vi "pump_test_backup.vi"() -> ()   [LabVIEW 2019]
uses:
  <vilib>/Instr/_visa.llb/VISA Configure Serial Port (Instr).vi
panel:
  in  "Frequency (%)":u16
  out "Error Out":errorcluster={"status"=FALSE, "code"=1073676294, "source"="VISA Read in pump_test.vi"}
  out "Time and torque":string="15.07.22\t0\r"
  in  "stop":bool
  out "Current readind (A)":dbl format="%.2g"
  out "Frequency reading (Hz)":dbl format="%.2g"
  out "Torque readind (%)":dbl
  out "Speed (km/h)":dbl format="%.2g"
  out "Case temp (ºC)":dbl=35.0 format="%#_6f"
  out "RPM":dbl
  out "Revolutions":dbl format="%.2f"
  out "Km":dbl format="%.3f"
  out "Calculated torque ( Nm)":dbl=nan format="%.3f"
  out "Calculated torque  (%)":dbl=nan
  out "Potencia (kW)":dbl format="%.2f"
  out "substring encoder 2":string
  in  "Control Buttons":enum32{"stop", "start", "send"}(radio)
  out "Consumption":dbl(graph)
  out "Case temp reading (ºC)":dbl(graph)=35.0
  out "Freq reading (%)":dbl(graph)
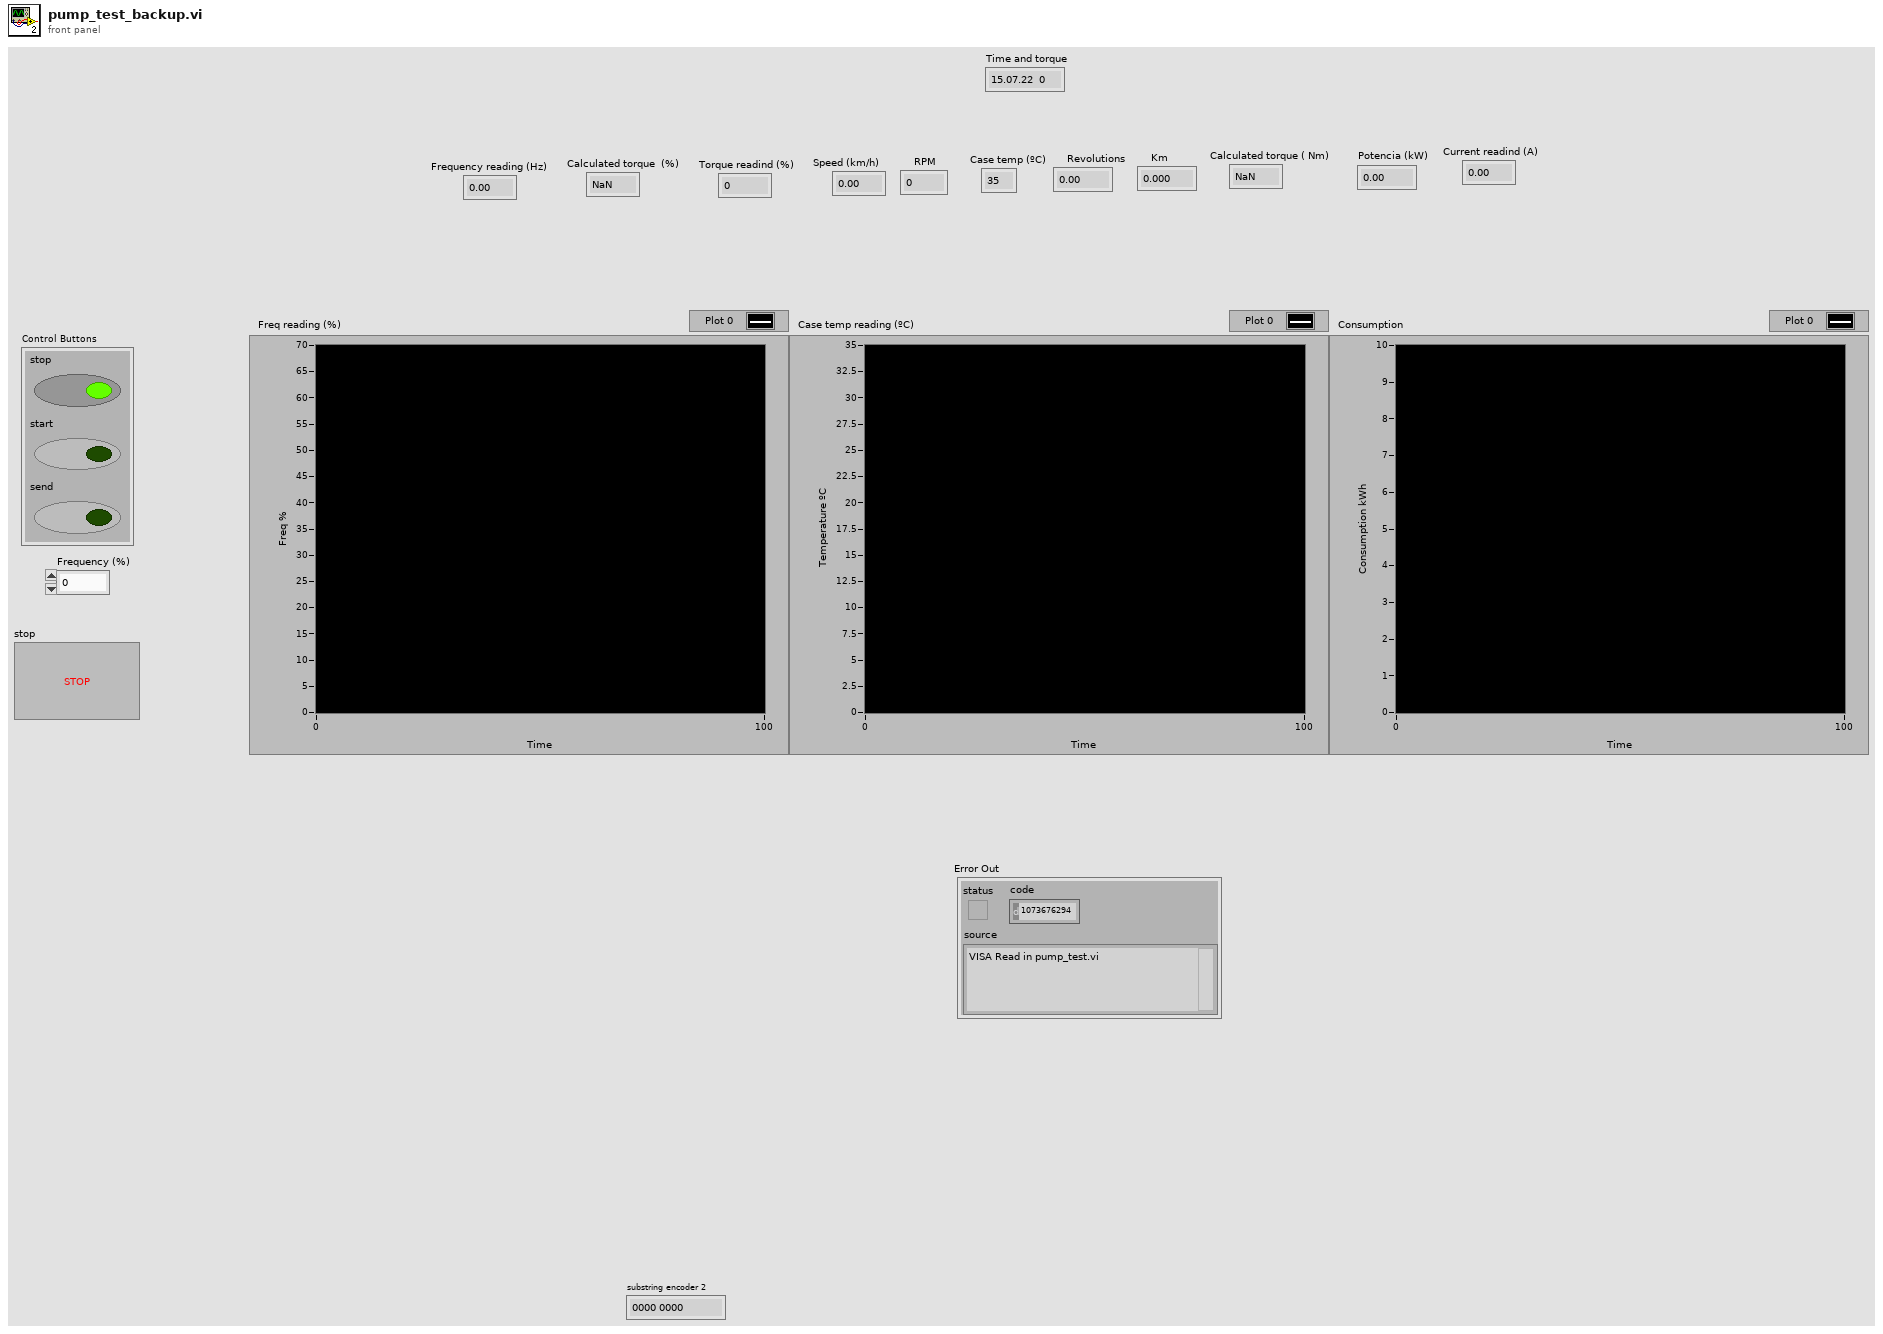
[diagram p1: front panel]
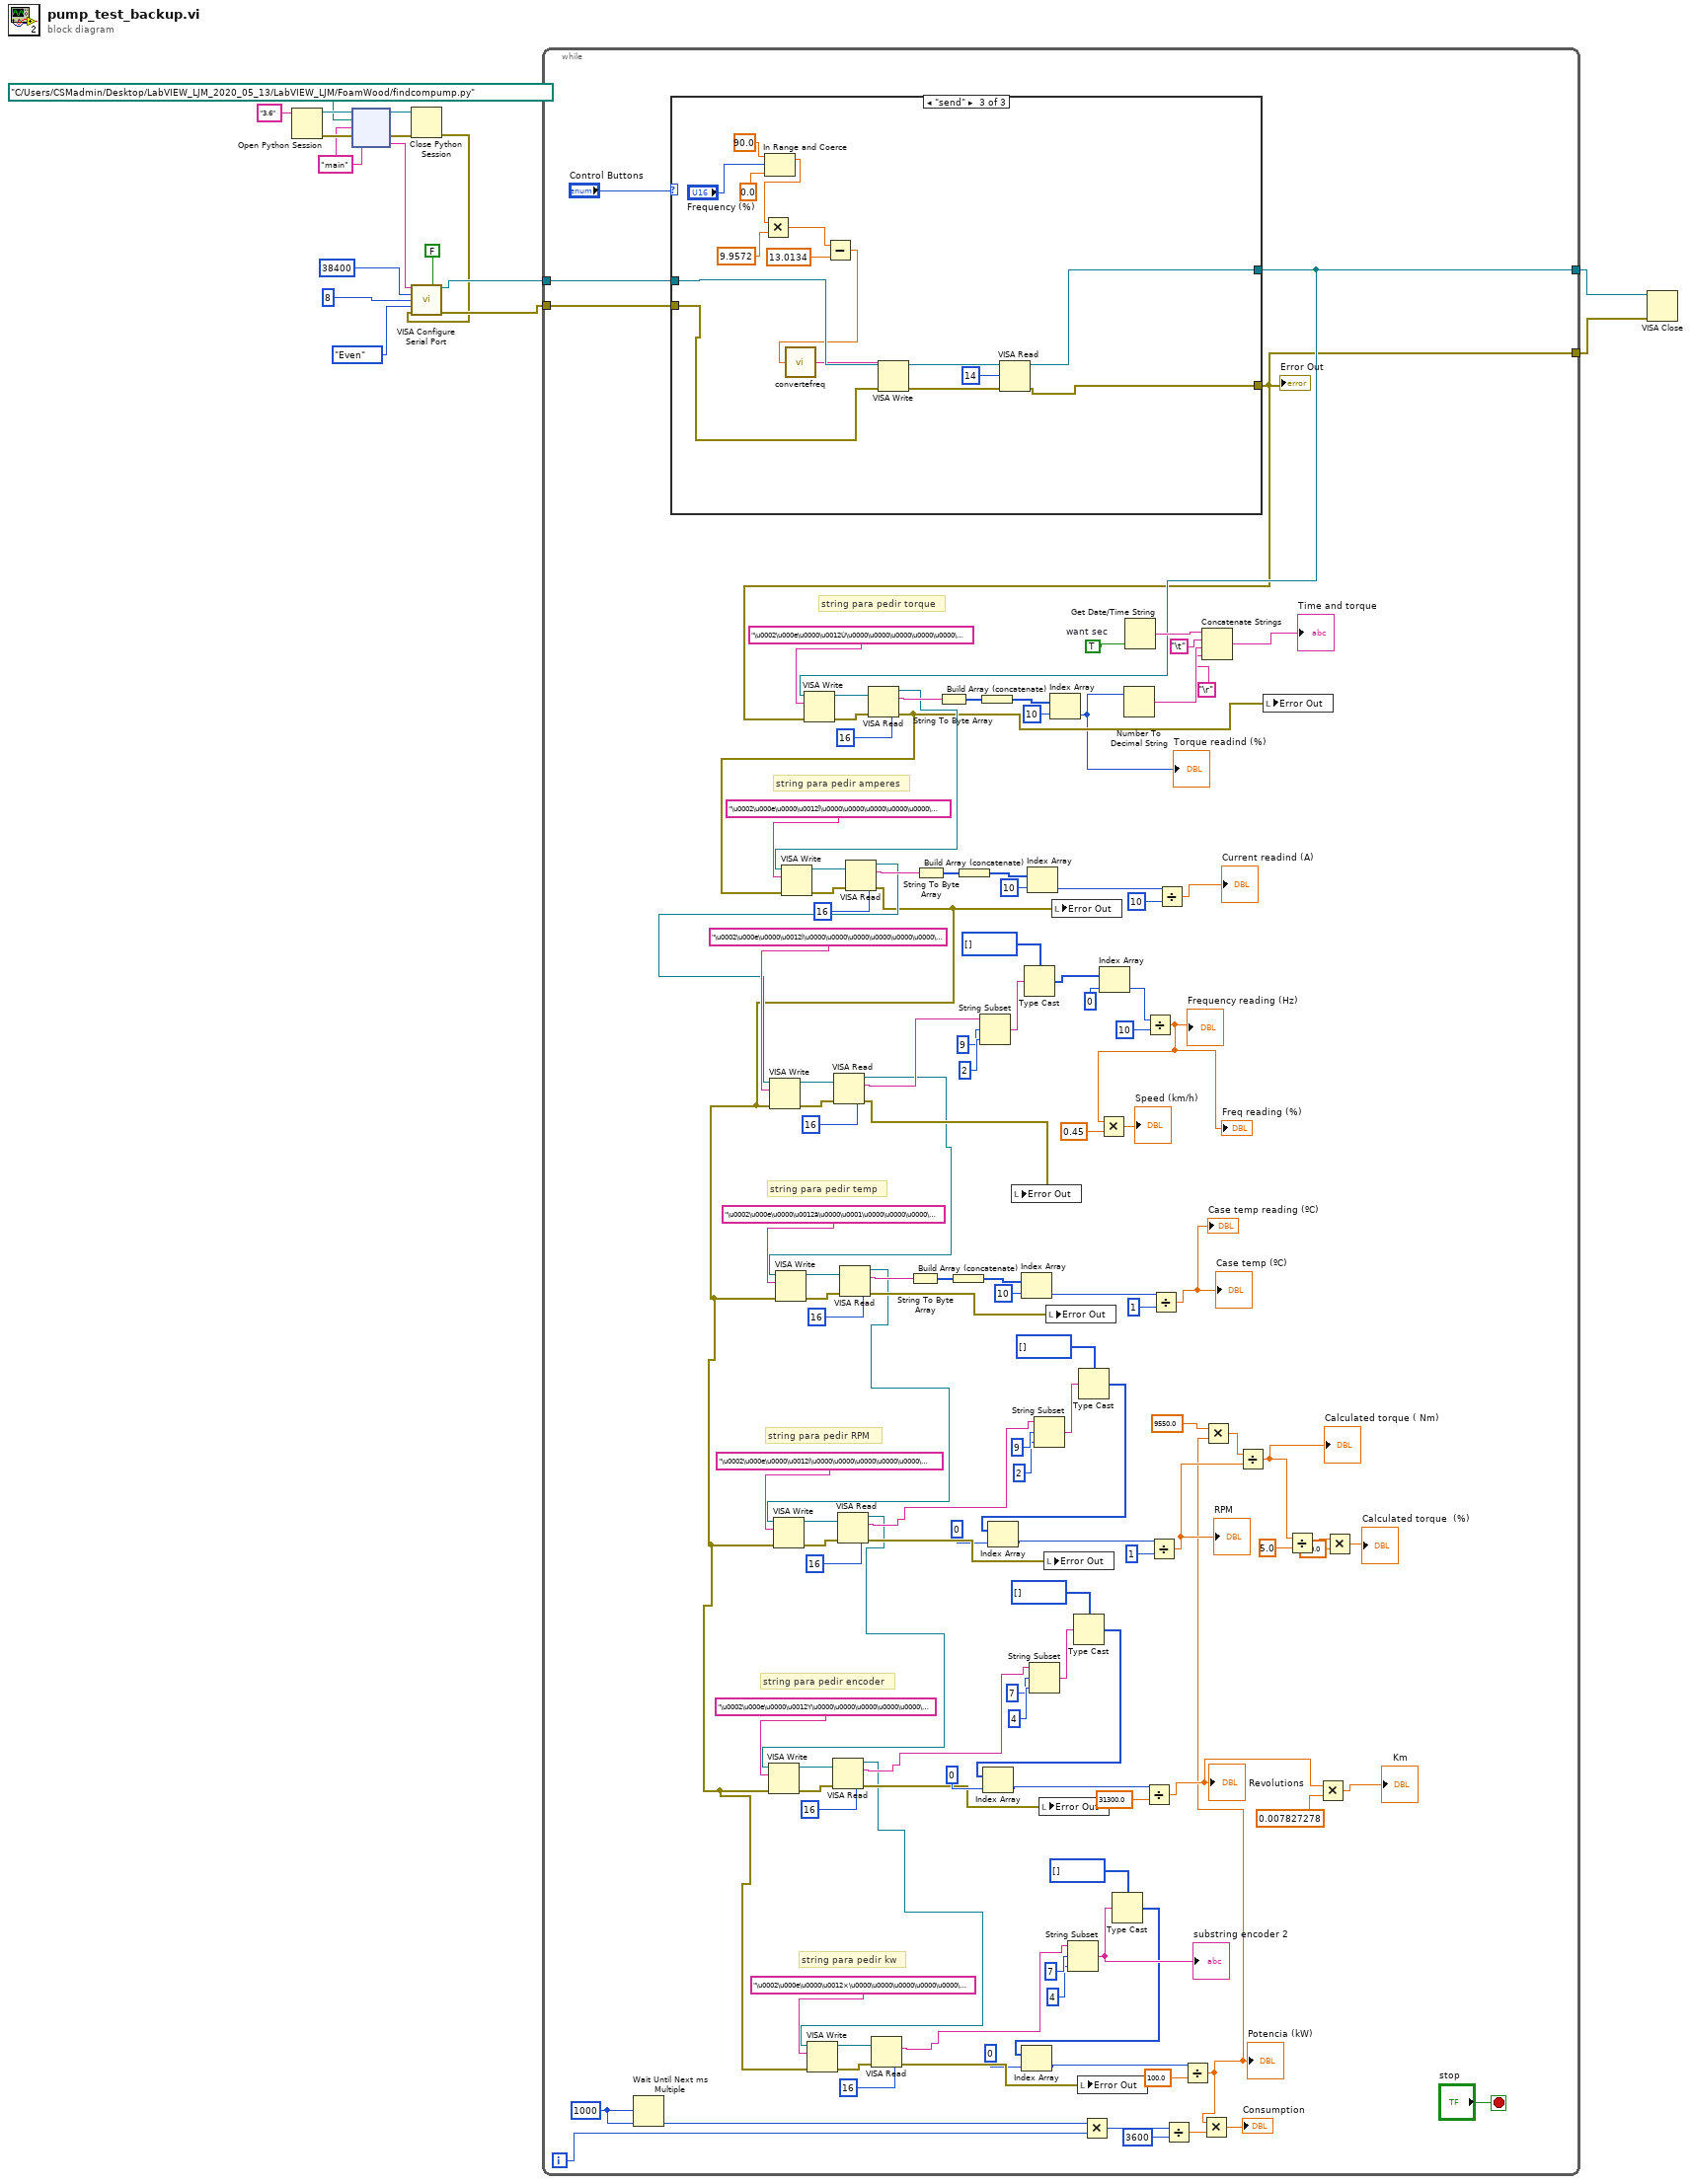
[diagram p0: block diagram]
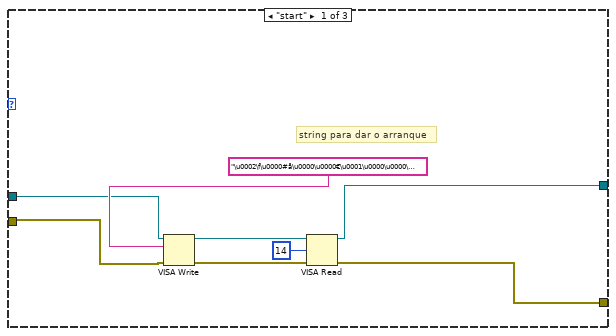
[diagram p2: hidden frame]
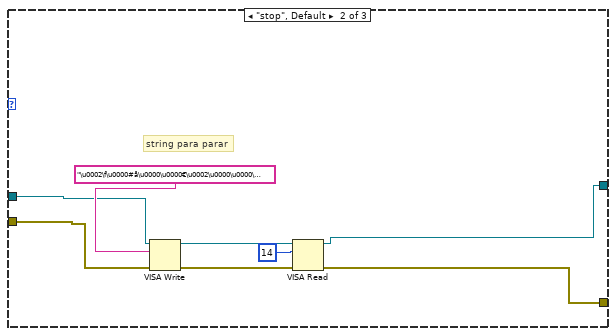
[diagram p3: hidden frame]
diagram:
  w11 = "main" ("function name")
  n1 = Open Python Session(python version="3.6" ("Python version")) -> (session out=w14:refnum<k35>, error out=w15:errorcluster)  [unwired: 2 in]
  n2 = node(w14, path "C:/Users/CSMadmin/Desktop/LabVIEW_LJM_2020_05_13/LabVIEW_LJM/FoamWood/findcompump.py" ("module path"), w11, w15, w11) -> (w3:refnum<k35>, w2:errorcluster, w8:string)  [unwired: 2 out]
  n3 = Close Python Session(session in=w3, error in=w2) -> (11:w1:errorcluster)
  n4 = call-poly "VISA Configure Serial Port"("VISA resource name"=w8, "Enable Termination\nChar (T)"=FALSE ("Enable Termination\nChar (T)"), "baud rate (9600)"=u32 38400, "data bits (8)"=u16 8, "parity (0:none)"=enum16{"None", "Odd", "Even", "Mark", "Space"}."Even", "error in (no error)"=w1) -> ("VISA resource name out"=w7:refnum<visa-resource-name>, "error out"=w6:errorcluster)  [unwired: 8 in]
  n5 = while {
    tunnel: w7 -> [w145]
    tunnel: w6 -> [w146]
    tunnel: [w129] -> w5
    tunnel: [w128] -> w4
    i -> [w24]
    stop <- "stop" stop-if-true
    w18 = u32 1000 ("millisecond multiple")
    w142 = TRUE  # want sec
    # "string para pedir kw"
    # "string para pedir encoder"
    # "string para pedir RPM"
    # "string para pedir temp"
    # "string para pedir amperes"
    # "string para pedir torque"
    n6 = Wait Until Next ms Multiple(millisecond multiple=w18) -> ()  [unwired: 1 out]
    n7 = case shown="\"send\"" "Control Buttons" {
      tunnel: w145 -> [w148 w161 w178]
      tunnel: w146 -> [w149 w160 w177]
      tunnel: [w153 w159 w176] -> w128
      tunnel: [w147 w155 w172] -> w129
      frame "start" {
        # "string para dar o arranque"
        n8 = VISA Write(VISA resource name=w148, write buffer="\u0002\f\u0000#å\u0000\u0000€\u0001\u0000\u0000\u0000\u0000I" ("write buffer (\"\")"), error in (no error)=w149) -> (VISA resource name out=w152:refnum<visa-resource-name>, error out=w150:errorcluster)  [unwired: 1 out]
        n9 = VISA Read(VISA resource name=w152, byte count=u32 14 ("Bytes to Read"), error in (no error)=w150) -> (VISA resource name out=w147:refnum<visa-resource-name>, error out=w153:errorcluster)  [unwired: 2 out]
      }
      frame "stop", Default {
        # "string para parar"
        n10 = VISA Write(VISA resource name=w161, write buffer="\u0002\f\u0000#å\u0000\u0000€\u0002\u0000\u0000\u0000\u0000J" ("write buffer (\"\")"), error in (no error)=w160) -> (VISA resource name out=w158:refnum<visa-resource-name>, error out=w156:errorcluster)  [unwired: 1 out]
        n11 = VISA Read(VISA resource name=w158, byte count=u32 14 ("Bytes to Read"), error in (no error)=w156) -> (VISA resource name out=w155:refnum<visa-resource-name>, error out=w159:errorcluster)  [unwired: 2 out]
      }
      frame "send" {
        n12 = In Range and Coerce(upper limit=90.0, x="Frequency (%)", lower limit=0.0) -> (coerced(x)=w164:dbl)  [unwired: 1 out]
        n13 = Multiply(x=w164, y=9.9572) -> (x*y=w168:dbl)
        n14 = Subtract(x=w168, y=13.0134) -> (x-y=w167:dbl)
        n15 = call "convertefreq.vi"("Numeric"=w167) -> ("string"=w171:string)
        n16 = VISA Write(VISA resource name=w178, write buffer=w171, error in (no error)=w177) -> (VISA resource name out=w175:refnum<visa-resource-name>, error out=w173:errorcluster)  [unwired: 1 out]
        n17 = VISA Read(VISA resource name=w175, byte count=u32 14 ("Bytes to Read"), error in (no error)=w173) -> (VISA resource name out=w172:refnum<visa-resource-name>, error out=w176:errorcluster)  [unwired: 2 out]
      }
    }
    "Error Out" <- w128
    n18 = VISA Write(VISA resource name=w129, write buffer="\u0002\u000e\u0000\u0012Ù\u0000\u0000\u0000\u0000\u0000\u0000\u0000\u0000\u0000\u0000Ç" ("write buffer (\"\")"), error in (no error)=w128) -> (VISA resource name out=w138:refnum<visa-resource-name>, error out=w139:errorcluster)  [unwired: 1 out]
    n19 = VISA Read(VISA resource name=w138, byte count=u32 16 ("Bytes to Read"), error in (no error)=w139) -> (VISA resource name out=w120:refnum<visa-resource-name>, read buffer=w132:string, error out=w119:errorcluster)  [unwired: 1 out]
    n20 = VISA Write(VISA resource name=w120, write buffer="\u0002\u000e\u0000\u0012Ï\u0000\u0000\u0000\u0000\u0000\u0000\u0000\u0000\u0000\u0000Ñ" ("write buffer (\"\")"), error in (no error)=w119) -> (VISA resource name out=w123:refnum<visa-resource-name>, error out=w122:errorcluster)  [unwired: 1 out]
    n21 = VISA Read(VISA resource name=w123, byte count=u32 16 ("Bytes to Read"), error in (no error)=w122) -> (VISA resource name out=w87:refnum<visa-resource-name>, read buffer=w109:string, error out=w33:errorcluster)  [unwired: 1 out]
    n22 = VISA Write(VISA resource name=w87, write buffer="\u0002\u000e\u0000\u0012Ì\u0000\u0000\u0000\u0000\u0000\u0000\u0000\u0000\u0000\u0000Ò" ("write buffer (\"\")"), error in (no error)=w33) -> (VISA resource name out=w111:refnum<visa-resource-name>, error out=w112:errorcluster)  [unwired: 1 out]
    n23 = VISA Read(VISA resource name=w111, byte count=u32 16 ("Bytes to Read"), error in (no error)=w112) -> (VISA resource name out=w79:refnum<visa-resource-name>, read buffer=w102:string, error out=w114:errorcluster)  [unwired: 1 out]
    n24 = VISA Write(VISA resource name=w79, write buffer="\u0002\u000e\u0000\u0012ã\u0000\u0001\u0000\u0000\u0000\u0000\u0000\u0000\u0000\u0000ü" ("write buffer (\"\")"), error in (no error)=w33) -> (VISA resource name out=w92:refnum<visa-resource-name>, error out=w93:errorcluster)  [unwired: 1 out]
    n25 = VISA Read(VISA resource name=w92, byte count=u32 16 ("Bytes to Read"), error in (no error)=w93) -> (VISA resource name out=w80:refnum<visa-resource-name>, read buffer=w97:string, error out=w98:errorcluster)  [unwired: 1 out]
    n26 = VISA Write(VISA resource name=w80, write buffer="\u0002\u000e\u0000\u0012Í\u0000\u0000\u0000\u0000\u0000\u0000\u0000\u0000\u0000\u0000Ó" ("write buffer (\"\")"), error in (no error)=w33) -> (VISA resource name out=w85:refnum<visa-resource-name>, error out=w84:errorcluster)  [unwired: 1 out]
    n27 = VISA Read(VISA resource name=w85, byte count=u32 16 ("Bytes to Read"), error in (no error)=w84) -> (VISA resource name out=w55:refnum<visa-resource-name>, read buffer=w74:string, error out=w81:errorcluster)  [unwired: 1 out]
    n28 = VISA Write(VISA resource name=w55, write buffer="\u0002\u000e\u0000\u0012Y\u0000\u0000\u0000\u0000\u0000\u0000\u0000\u0000\u0000\u0000G" ("write buffer (\"\")"), error in (no error)=w33) -> (VISA resource name out=w57:refnum<visa-resource-name>, error out=w58:errorcluster)  [unwired: 1 out]
    n29 = VISA Read(VISA resource name=w57, byte count=u32 16 ("Bytes to Read"), error in (no error)=w58) -> (VISA resource name out=w34:refnum<visa-resource-name>, read buffer=w66:string, error out=w61:errorcluster)  [unwired: 1 out]
    n30 = VISA Write(VISA resource name=w34, write buffer="\u0002\u000e\u0000\u0012×\u0000\u0000\u0000\u0000\u0000\u0000\u0000\u0000\u0000\u0000É" ("write buffer (\"\")"), error in (no error)=w33) -> (VISA resource name out=w46:refnum<visa-resource-name>, error out=w45:errorcluster)  [unwired: 1 out]
    n31 = VISA Read(VISA resource name=w46, byte count=u32 16 ("Bytes to Read"), error in (no error)=w45) -> (read buffer=w32:string, error out=w42:errorcluster)  [unwired: 2 out]
    n32 = String To Byte Array(string=w97) -> (unsigned byte array=w90:u8[])
    n33 = String To Byte Array(string=w109) -> (unsigned byte array=w125:u8[])
    n34 = String To Byte Array(string=w132) -> (unsigned byte array=w136:u8[])
    n35 = Build Array (concatenate)(w90) -> (w89:u8[])
    n36 = Build Array (concatenate)(w125) -> (w126:u8[])
    n37 = String Subset(string=w102, offset (0)=9, length (rest)=2 ("length (rest)")) -> (substring=w101:string)
    n38 = Build Array (concatenate)(w136) -> (w135:u8[])
    n39 = local write "Error Out"(w114) -> ()
    n40 = Index Array(array=w89, index=10) -> (element=w95:u8)
    n41 = Type Cast(type=u16[] [], x=w101) -> (*(type *) &x=w100:u16[])
    n42 = Index Array(array=w126, index=10) -> (element=w118:u8)
    n43 = String Subset(string=w66, offset (0)=7, length (rest)=4 ("length (rest)")) -> (substring=w63:string)
    n44 = String Subset(string=w74, offset (0)=9, length (rest)=2 ("length (rest)")) -> (substring=w77:string)
    n45 = local write "Error Out"(w61) -> ()
    n46 = local write "Error Out"(w81) -> ()
    n47 = local write "Error Out"(w98) -> ()
    n48 = Index Array(array=w135, index=10) -> (element=w70:u8)
    "Torque readind (%)" <- w70
    n49 = local write "Error Out"(w33) -> ()
    n50 = String Subset(string=w32, offset (0)=7, length (rest)=4 ("length (rest)")) -> (substring=w40:string)
    "substring encoder 2" <- w40
    n51 = Type Cast(type=i32[] [], x=w63) -> (*(type *) &x=w68:i32[])
    n52 = Index Array(array=w68, index=0) -> (element=w69:i32)
    n53 = local write "Error Out"(w42) -> ()
    n54 = Type Cast(type=u16[] [], x=w77) -> (*(type *) &x=w72:u16[])
    n55 = Index Array(array=w72, index=0) -> (element=w71:u16)
    n56 = Multiply(x=w18, y=w24) -> (x*y=w22:u32)
    n57 = Index Array(array=w100, index=0) -> (element=w105:u16)
    n58 = Type Cast(type=i32[] [], x=w40) -> (*(type *) &x=w36:i32[])
    n59 = Index Array(array=w36, index=0) -> (element=w35:i32)
    n60 = Number To Decimal String(number=w70) -> (decimal integer string=w140:string)  [unwired: 1 in]
    n61 = Get Date/Time String(want seconds? (F)=w142) -> (time string=w143:string)  [unwired: 2 in, 1 out]
    n62 = Divide(x=w69, y=31300.0) -> (x/y=w54:dbl)
    "Revolutions" <- w54
    n63 = Divide(x=w105, y=u8 10) -> (x/y=w26:dbl)
    "Frequency reading (Hz)" <- w26
    "Freq reading (%)" <- w26
    n64 = Multiply(x=w26, y=0.45) -> (x*y=→"Speed (km/h)":dbl)
    n65 = Divide(x=w71, y=u8 1) -> (x/y=w25:dbl)
    "RPM" <- w25
    n66 = Divide(x=w95, y=u8 1) -> (x/y=→"Case temp (ºC)" →"Case temp reading (ºC)":dbl)
    n67 = Divide(x=w118, y=u8 10) -> (x/y=→"Current readind (A)":dbl)
    n68 = Divide(x=w22, y=u32 3600) -> (x/y=w20:dbl)
    n69 = Divide(x=w35, y=100.0) -> (x/y=w23:dbl)
    "Potencia (kW)" <- w23
    n70 = Multiply(x=w23, y=w20) -> (x*y=→"Consumption":dbl)
    n71 = Concatenate Strings(w143, "\t" ("Tab"), w140, "\r") -> (→"Time and torque":string)
    n72 = Multiply(x=9550.0, y=w23) -> (x*y=w30:dbl)
    n73 = Divide(x=w30, y=w25) -> (x/y=w29:dbl)
    "Calculated torque ( Nm)" <- w29
    n74 = local write "Error Out"(w119) -> ()
    n75 = Divide(x=w29, y=5.0) -> (x/y=w50:dbl)
    n76 = Multiply(x=w54, y=0.007827278) -> (x*y=→"Km":dbl)
    n77 = Multiply(x=w50, y=100.0) -> (x*y=→"Calculated torque  (%)":dbl)
  }
  n78 = VISA Close(VISA resource name=w5, error in (no error)=w4) -> ()  [unwired: 1 out]
